vi "Set Property.vi"(8 "error in (no error)":errorcluster, 9 "Value":dbl, 10 "Property":string, 11 "FM Sweep in":refnum<class "FM Sweep.lvclass">) -> (0 "error out":errorcluster, 3 "FM Sweep out":refnum<class "FM Sweep.lvclass">)   [LabVIEW 2020, in "FM Sweep.lvclass"]
uses:
  FM Sweep.lvclass
  FM Sweep.lvclass/FM Sweep.ctl
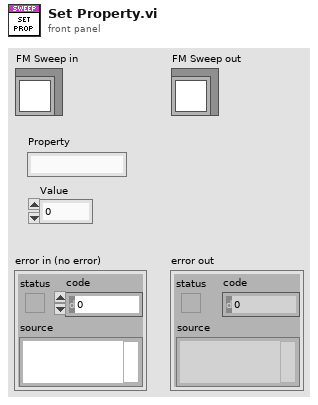
[diagram p1: front panel]
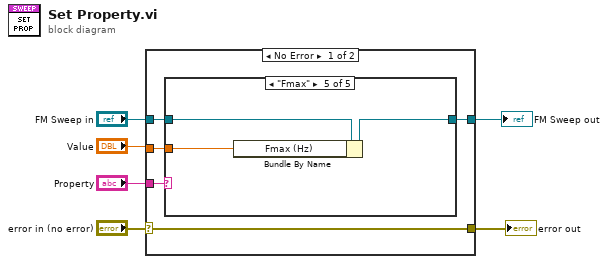
[diagram p0: block diagram]
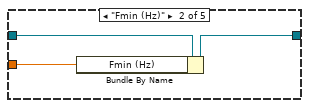
[diagram p3: hidden frame]
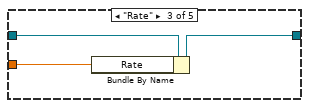
[diagram p4: hidden frame]
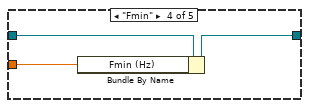
[diagram p5: hidden frame]
diagram:
  n1 = case shown="No Error" "error in (no error)" {
    selector: "error in (no error)" -> [w11 w25]
    tunnel: [w11 w25] -> w4
    tunnel: "Property" -> [w10 _]
    tunnel: "FM Sweep in" -> [w9 w26]
    tunnel: "Value" -> [w8 _]
    tunnel: [w7 w26] -> w3
    frame No Error {
      n2 = case shown="\"Fmax\"" w10 {
        tunnel: w9 -> [w12 w15 w18 w21 w24]
        tunnel: w8 -> [_ w14 w17 w20 w23]
        tunnel: [w12 w13 w16 w19 w22] -> w7
        frame "", Default {
        }
        frame "Fmin (Hz)" {
          n3 = Bundle By Name(cluster=w15, "Fmin (Hz)"=w14) -> (w13:refnum<class "FM Sweep.lvclass">)
        }
        frame "Rate" {
          n4 = Bundle By Name(cluster=w18, "Rate"=w17) -> (w16:refnum<class "FM Sweep.lvclass">)
        }
        frame "Fmin" {
          n5 = Bundle By Name(cluster=w21, "Fmin (Hz)"=w20) -> (w19:refnum<class "FM Sweep.lvclass">)
        }
        frame "Fmax" {
          n6 = Bundle By Name(cluster=w24, "Fmax (Hz)"=w23) -> (w22:refnum<class "FM Sweep.lvclass">)
        }
      }
    }
    frame Error {
    }
  }
  "error out" <- w4
  "FM Sweep out" <- w3
